vi "Variant to Tree.vi"(11 "?":variant) -> (2 "Value String":string, 3 "Boolean":bool)   [LabVIEW 2017]
uses:
  DSF Configuration Utility.lvlib
panel:
  in  "Tree":string(tree)
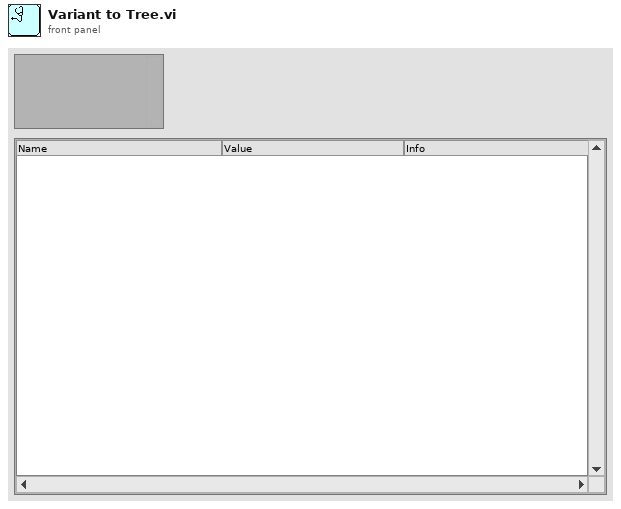
[diagram p1: front panel]
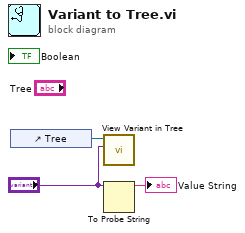
[diagram p0: block diagram]
diagram:
  n1 = control-ref of="Tree"() -> (w1:refnum<vi>)
  n2 = call "View Variant in Tree.vi"("Variant"="?", "TreeControl in"=w1) -> ()  [unwired: 9 in, 1 out]
  n3 = To Probe String(7:"?") -> (3:→"Value String":string)  [unwired: 2 in, 1 out]
